vi "removeFormatting.vi"(8 "error in (no error)":errorcluster, 10 "input":string, 11 "XMLPrettyPrinting in":refnum<class "XMLPrettyPrinting.lvclass">) -> (0 "error out":errorcluster, 2 "output":string, 3 "XMLPrettyPrinting out":refnum<class "XMLPrettyPrinting.lvclass">)   [LabVIEW 2011, in "Views.lvlib" / "ViewerTools.lvlib" / "XMLPrettyPrinting.lvclass"]
uses:
  XMLPrettyPrinting.lvclass
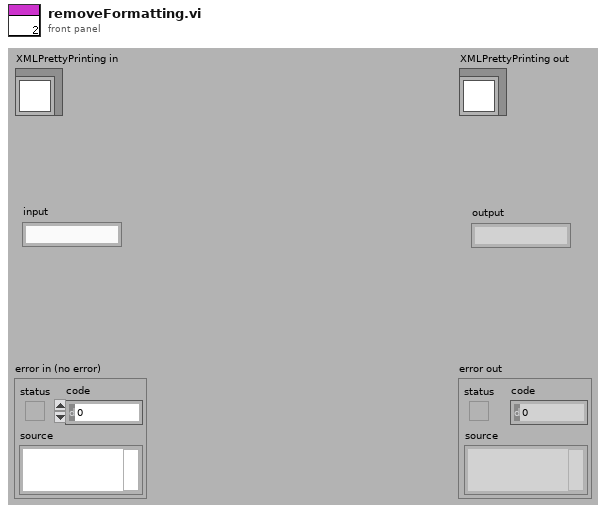
[diagram p1: front panel]
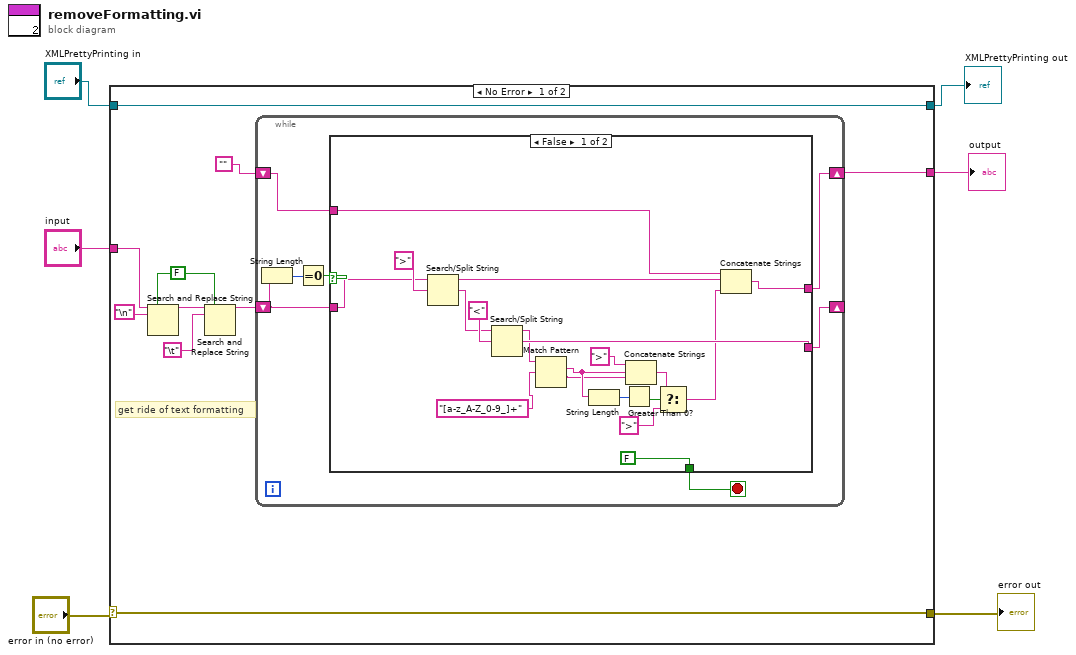
[diagram p0: block diagram]
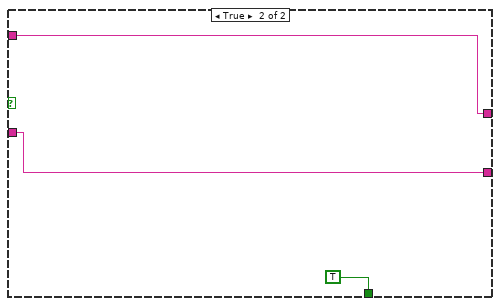
[diagram p2: hidden frame]
diagram:
  n1 = case shown="No Error" "error in (no error)" {
    selector: "error in (no error)" -> [w8 w47]
    tunnel: [w10 _] -> w6
    tunnel: "XMLPrettyPrinting in" -> [w9 w46]
    tunnel: [w9 w46] -> w3
    tunnel: [w8 w47] -> w2
    tunnel: "input" -> [w7 _]
    frame No Error {
      w15 = FALSE
      # "get ride of text formatting"
      n2 = Search and Replace String(replace all?=w15, input string=w7, search string="\n") -> (result string=w14:string)  [unwired: 5 in, 3 out]
      n3 = Search and Replace String(replace all?=w15, input string=w14, search string="\t") -> (result string=w12:string)  [unwired: 5 in, 3 out]
      n4 = while {
        shift-right: [w19] -> _
        shift-left: w12 -> [w22]
        shift-right: [w18] -> w10
        shift-left: "" -> [w17]
        stop <- w20 stop-if-true
        n5 = String Length(string=w22) -> (length=w23:i32)
        n6 = Equal To 0?(x=w23) -> (x = 0?=w21:bool)
        n7 = case shown="False" w21 {
          tunnel: w22 -> [w24 w43]
          tunnel: [FALSE TRUE] -> w20
          tunnel: [w41 w44] -> w18
          tunnel: [w40 w43] -> w19
          tunnel: w17 -> [w39 w44]
          frame False {
            n8 = Search/Split String(string=w24, search string/char (-)=">") -> (substring before match=w31:string, match + rest of string=w28:string)  [unwired: 1 in, 1 out]
            n9 = Search/Split String(string=w28, search string/char (-)="<") -> (substring before match=w27:string, match + rest of string=w40:string)  [unwired: 1 in, 1 out]
            n10 = Match Pattern(string=w27, regular expression="[a-z_A-Z_0-9_]+") -> (match substring=w35:string, after substring=w34:string)  [unwired: 1 in, 2 out]
            n11 = String Length(string=w35) -> (length=w36:i32)
            n12 = Greater Than 0?(x=w36) -> (x > 0?=w33:bool)
            n13 = Concatenate Strings(">", w35, w34) -> (w32:string)
            n14 = Select(t=w32, s=w33, f=">") -> (s? t:f=w30:string)
            n15 = Concatenate Strings(w39, w31, w30) -> (w41:string)
          }
          frame True {
          }
        }
      }
    }
    frame Error {
    }
  }
  "error out" <- w2
  "XMLPrettyPrinting out" <- w3
  "output" <- w6
